vi "GUI TWM setup.vi"(11 "TWM pipe":string="\\\\.\\pipe\\TWM:server") -> (3 "TWM pipe out":string)   [LabVIEW 2020]
doc: "Use this template to build a producer/consumer design pattern with events to produce queue items. Use this design pattern instead of the User Interface Event Handler pattern for user interfaces when you want to execute code asynchronously in response to an event without slowing the user interface responsiveness."
uses:
  <vilib>/Utility/error.llb/DialogType.ctl
  <vilib>/Utility/error.llb/Error Cluster From Error Code.vi
  <vilib>/ErrorRing/Error Ring.xnode
  external libraries/varilib/varilib.lvlib
  external libraries/TWM client.lvlibp
  external libraries/QuPMXLabVIEWdriver/QuPMXdriver.lvlib
panel:
  in  "mx control":bool
  in  "make_corrections":bool
  out "gui_elements":refnum<vi>[](array[refnum])
  out "Status":string
  in  "save_and_quit":bool
  in  "test":bool
  in  "cancel":bool
  # "You must set following in TWM according your setup:\n1, Octave/Matlab\n2, Digitizers\n   If using 3458, set Aperture mode to Auto\n   If using 5922, disable streaming mode,\n                            set 10 MHz reference if available\n3, Multiplexer\n4, Measurement configuration:\n                            folder,\n                            filename,\n                            comment,\n                            etc."
  # "QPSCONTROL changes only following in the TWM:\n1, Sampling rage (TWM->Setup Measurement)\n2, Samples count (TWM->Setup Measurement)\n3, Records count (TWM->Setup Measurement)\n4, Sub-records count (TWM->Setup Measurement)\n5, Trigger (mode, source, level, coupling\n                                     (TWM->Setup Measurment)"
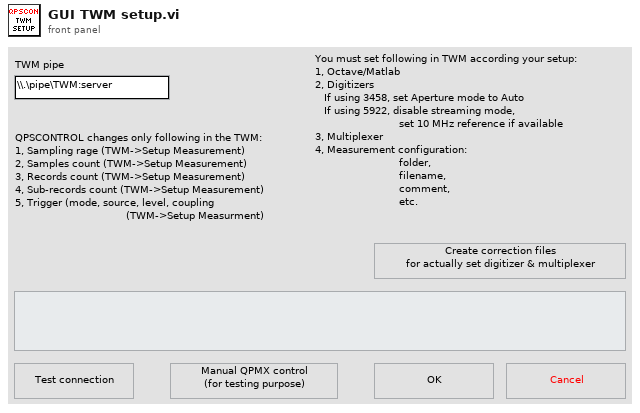
[diagram p1: front panel]
types:
  T1 = typedef "DialogType.ctl" = u16
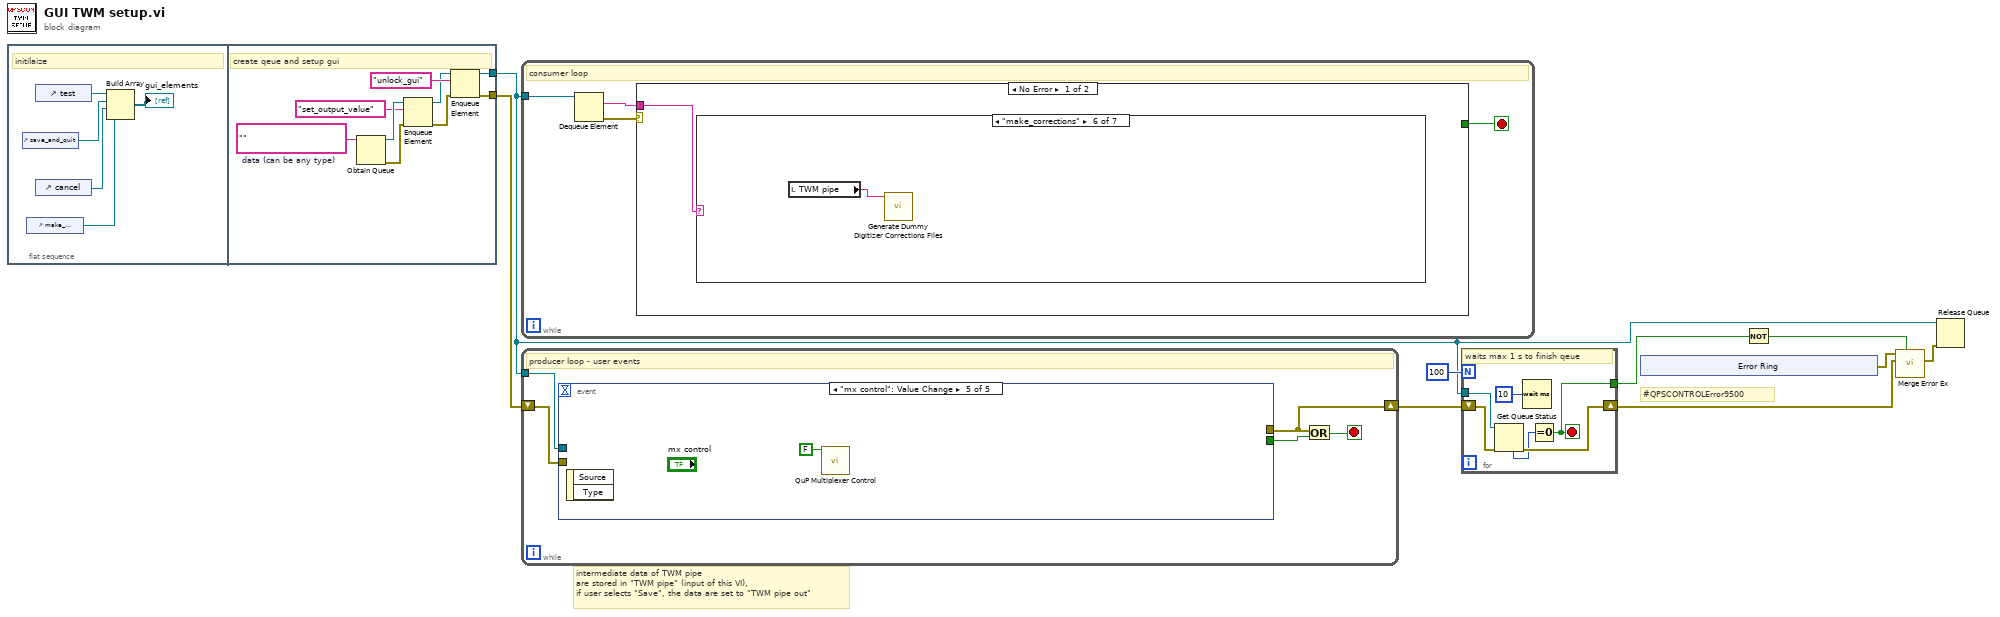
[diagram p0: block diagram]
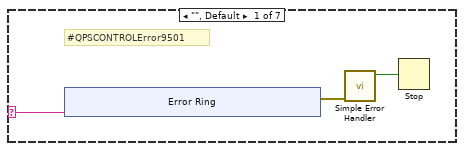
[diagram p2: hidden frame]
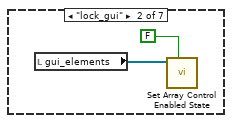
[diagram p3: hidden frame]
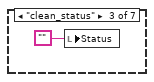
[diagram p4: hidden frame]
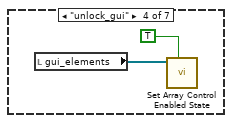
[diagram p5: hidden frame]
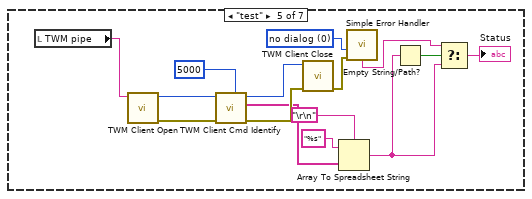
[diagram p6: hidden frame]
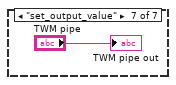
[diagram p7: hidden frame]
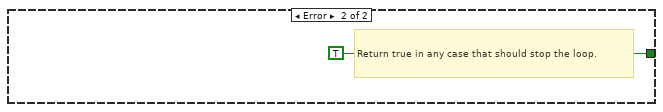
[diagram p8: hidden frame]
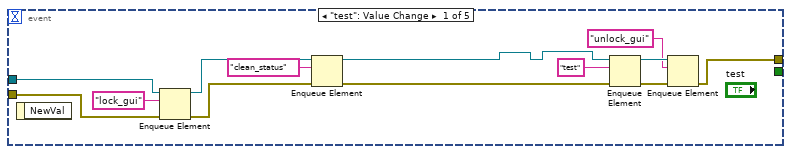
[diagram p9: hidden frame]
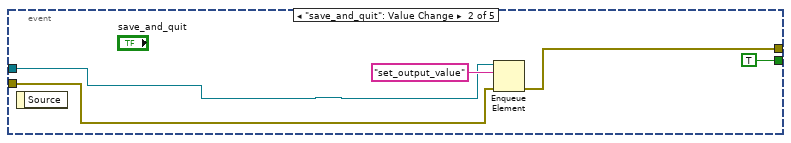
[diagram p10: hidden frame]
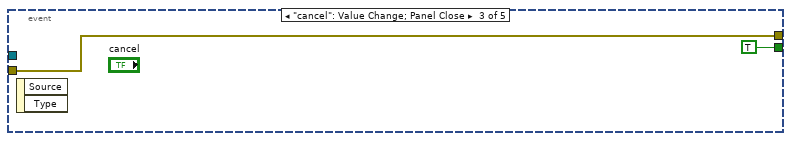
[diagram p11: hidden frame]
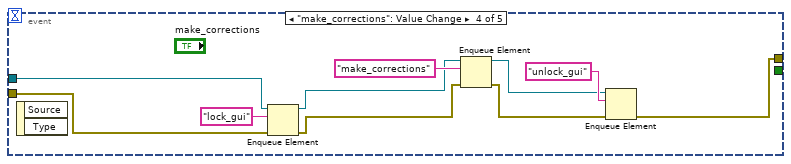
[diagram p12: hidden frame]
diagram:
  # "#QPSCONTROLError9500"
  # "intermediate data of TWM pipe\nare stored in \"TWM pipe\" (input of this VI),\nif user selects \"Save\", the data are set to \"TWM pipe out\""
  n1 = flat-sequence {
    tunnel: [w19] -> w2
    tunnel: [w17] -> w1
    frame #0 {
      # "initilaize"
      n2 = control-ref of="save_and_quit"() -> (w13:refnum<vi>)
      n3 = control-ref of="make_corrections"() -> (w10:refnum<vi>)
      n4 = control-ref of="test"() -> (w14:refnum<vi>)
      n5 = control-ref of="cancel"() -> (w12:refnum<vi>)
      n6 = Build Array(w14, w13, w12, w10) -> (→"gui_elements":refnum<vi>[])
    }
    frame #1 {
      w18 = ""  # data (can be any type)
      # "create qeue and setup gui"
      n7 = Obtain Queue(element data type=w18) -> (queue out=w22:refnum<queue>, error out=w23:errorcluster)  [unwired: 4 in, 1 out]
      n8 = Enqueue Element(queue=w22, element="set_output_value", error in (no error)=w23) -> (queue out=w15:refnum<queue>, error out=w16:errorcluster)  [unwired: 1 in, 1 out]
      n9 = Enqueue Element(queue=w15, element="unlock_gui", error in (no error)=w16) -> (queue out=w19:refnum<queue>, error out=w17:errorcluster)  [unwired: 1 in, 1 out]
    }
  }
  n10 = while {
    tunnel: w2 -> [w27]
    stop <- w24 stop-if-true
    # "consumer loop"
    n11 = Dequeue Element(queue=w27) -> (element=w25:string, error out=w26:errorcluster)  [unwired: 2 in, 2 out]
    n12 = case shown="No Error" w26 {
      tunnel: w25 -> [w28 _]
      tunnel: [_ TRUE] -> w24
      frame No Error {
        n13 = case shown="\"make_corrections\"" w28 {
          selector: w28 -> [w29 _ _ _ _ _ _]
          frame "", Default {
            # "#QPSCONTROLError9501"
            n14 = xnode "Error Ring"("parameter 0"=w29) -> ("error out"=w31:errorcluster)
            n15 = call <vilib>:"Simple Error Handler.vi"("error in (no error)"=w31) -> ("error?"=w30:bool)  [unwired: 4 in, 4 out]
            n16 = Stop(stop? (T)=w30) -> ()
          }
          frame "lock_gui" {
            n17 = local read "gui_elements"() -> (w40:refnum<vi>[])
            n18 = call "Set Array Control Enabled State.vi"("enabled (T)"=FALSE, "reference array in"=w40) -> ()  [unwired: 8 in, 2 out]
          }
          frame "clean_status" {
            n19 = local write "Status"("") -> ()
          }
          frame "unlock_gui" {
            n20 = local read "gui_elements"() -> (w43:refnum<vi>[])
            n21 = call "Set Array Control Enabled State.vi"("enabled (T)"=TRUE, "reference array in"=w43) -> ()  [unwired: 8 in, 2 out]
          }
          frame "test" {
            w49 = T1 0 items=["no dialog", "OK message", "continue or stop message", "OK message + warnings", "continue/stop + warnings"] ("type of dialog (OK msg:1)")
            n22 = local read "TWM pipe"() -> (w45:string)
            n23 = call "TWM Client Open.vi"("pipe name"=w45) -> ("error out"=w57:errorcluster, "handle out"=w56:i32)  [unwired: 9 in]
            n24 = call "TWM Client Cmd Identify.vi"("timeout [ms]"=5000, "error in"=w57, "handle"=w56) -> ("error out"=w58:errorcluster, "channel idns"=w53:string[], "handle out"=w55:i32)  [unwired: 5 in, 1 out]
            n25 = call "TWM Client Close.vi"("error in"=w58, "handle in"=w55) -> ("error out"=w50:errorcluster)  [unwired: 9 in]
            n26 = Array To Spreadsheet String(delimiter (Tab)="\r\n", array=w53, 3:"%s" ("format string")) -> (spreadsheet string=w46:string)
            n27 = call <vilib>:"Simple Error Handler.vi"("type of dialog (OK msg:1)"=w49, "error in (no error)"=w50) -> ("message"=w47:string)  [unwired: 3 in, 4 out]
            n28 = Empty String/Path?(string/path=w46) -> (empty?=w48:bool)
            n29 = Select(t=w47, s=w48, f=w46) -> (s? t:f=→"Status":string)
          }
          frame "make_corrections" {
            n30 = local read "TWM pipe"() -> (w59:string)
            n31 = call "Generate Dummy Digitizer Corrections Files.vi"("TWM pipe"=w59) -> ()  [unwired: 10 in, 1 out]
          }
          frame "set_output_value" {
            "TWM pipe out" <- "TWM pipe"
          }
        }
      }
      frame Error {
        # "Return true in any case that should stop the loop."
      }
    }
  }
  n32 = while {
    shift-right: [w62] -> w5
    shift-left: w1 -> [w65]
    tunnel: w2 -> [w66]
    stop <- w63 stop-if-true
    # "producer loop - user events"
    n33 = event shown="[4] \"mx control\": Value Change" {
      selector: _ -> [_ _ _ _ _]
      dyn-events: _ -> [_ _ _ _ _]
      timeout: _ -> [_ _ _ _ _]
      tunnel: w66 -> [w73 w81 _ w93 _]
      tunnel: w65 -> [w74 w80 w86 w92 _]
      tunnel: [w77 w82 w86 w87 _] -> w62
      tunnel: [_ TRUE ("cancel") TRUE ("cancel") _ _] -> w64
      event "test": Value Change {
        n34 = event-data() -> ()  [unwired: 1 in, 1 out]
        n35 = Enqueue Element(queue=w73, element="lock_gui", error in (no error)=w74) -> (queue out=w70:refnum<queue>, error out=w71:errorcluster)  [unwired: 1 in, 1 out]
        n36 = Enqueue Element(queue=w70, element="clean_status", error in (no error)=w71) -> (queue out=w68:refnum<queue>, error out=w67:errorcluster)  [unwired: 1 in, 1 out]
        n37 = Enqueue Element(queue=w68, element="test", error in (no error)=w67) -> (queue out=w76:refnum<queue>, error out=w78:errorcluster)  [unwired: 1 in, 1 out]
        n38 = Enqueue Element(queue=w76, element="unlock_gui", error in (no error)=w78) -> (error out=w77:errorcluster)  [unwired: 1 in, 2 out]
      }
      event "save_and_quit": Value Change {
        n39 = event-data() -> ()  [unwired: 1 in, 1 out]
        n40 = Enqueue Element(queue=w81, element="set_output_value", error in (no error)=w80) -> (error out=w82:errorcluster)  [unwired: 1 in, 2 out]
      }
      event "cancel": Value Change; Panel Close {
        n41 = event-data() -> ()  [unwired: 1 in, 2 out]
      }
      event "make_corrections": Value Change {
        n42 = event-data() -> ()  [unwired: 1 in, 2 out]
        n43 = Enqueue Element(queue=w93, element="lock_gui", error in (no error)=w92) -> (queue out=w90:refnum<queue>, error out=w91:errorcluster)  [unwired: 1 in, 1 out]
        n44 = Enqueue Element(queue=w90, element="make_corrections", error in (no error)=w91) -> (queue out=w88:refnum<queue>, error out=w89:errorcluster)  [unwired: 1 in, 1 out]
        n45 = Enqueue Element(queue=w88, element="unlock_gui", error in (no error)=w89) -> (error out=w87:errorcluster)  [unwired: 1 in, 2 out]
      }
      event "mx control": Value Change {
        n46 = event-data() -> ()  [unwired: 1 in, 2 out]
        n47 = call "QuP Multiplexer Control.vi"("Do full quit? (T)"=FALSE) -> ()  [unwired: 11 in]
      }
    }
    n48 = Or(x=w62, y=w64) -> (x .or. y?=w63:bool)
  }
  n49 = for {
    N: 100 -> [_]
    tunnel: w2 -> [w103]
    shift-right: [w101] -> w6
    shift-left: w5 -> [w102]
    tunnel: [w98] -> w3
    stop <- w98 stop-if-true
    # "waits max 1 s to finish qeue"
    n50 = Get Queue Status(queue=w103, error in (no error)=w102) -> (error out=w101:errorcluster, # elements in queue=w99:i32)  [unwired: 1 in, 6 out]
    n51 = Wait (ms)(milliseconds to wait=u32 10) -> ()  [unwired: 1 out]
    n52 = Equal To 0?(x=w99) -> (x = 0?=w98:bool)
  }
  n53 = xnode "Error Ring"() -> ("error out"=w7:errorcluster)
  n54 = Not(x=w3) -> (.not. x?=w8:bool)
  n55 = call "Merge Error Ex.vi"("Is error? (False)"=w8, "main error in (no error)"=w6, "second error in"=w7) -> ("error out"=w4:errorcluster)  [unwired: 8 in]
  n56 = Release Queue(queue=w2, error in (no error)=w4) -> ()  [unwired: 1 in, 3 out]
